vi "write_attributes.vi"(8 "error in (no error)":errorcluster caption="entrée d'erreur (pas d'erreur)", 10 "attributes":T1, 11 "TSNE en entrée":refnum<class "TSNE.lvclass">) -> (0 "error out":errorcluster caption="sortie d'erreur", 3 "TSNE en sortie":refnum<class "TSNE.lvclass">)   [LabVIEW 2020, in "TSNE.lvclass"]
uses:
  TSNE.lvclass
  Controls/tsne_attributes.ctl
  TSNE.lvclass/TSNE.ctl
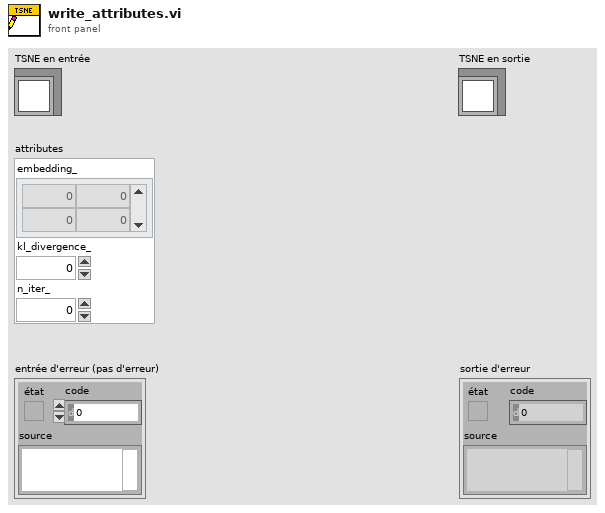
[diagram p1: front panel]
types:
  T1 = typedef "tsne_attributes.ctl" = cluster{"embedding_":dbl[][], "kl_divergence_":dbl, "n_iter_":dbl}
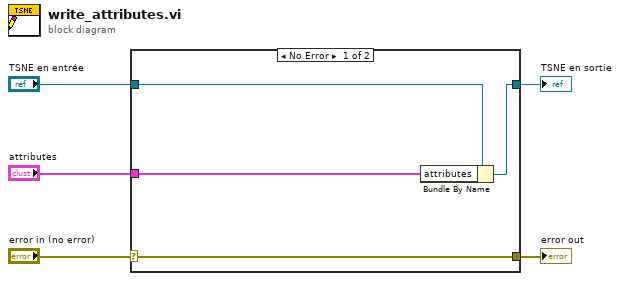
[diagram p0: block diagram]
diagram:
  n1 = case shown="No Error" "error in (no error)" {
    selector: "error in (no error)" -> [w9 w10]
    tunnel: [w9 w10] -> w4
    tunnel: [w7 w11] -> w2
    tunnel: "TSNE en entrée" -> [w8 w11]
    tunnel: "attributes" -> [w6 _]
    frame No Error {
      n2 = Bundle By Name(cluster=w8, "attributes"=w6) -> (w7:refnum<class "TSNE.lvclass">)
    }
    frame Error {
    }
  }
  "error out" <- w4
  "TSNE en sortie" <- w2
